vi "Send_picture.vi"() -> ()   [LabVIEW 2018]
uses:
  <vilib>/myRIO/Instrument Drivers/Onboard IO/UART/typedef/VISA Configuration.ctl
  <vilib>/Instr/_visa.llb/VISA Configure Serial Port (Instr).vi
  <vilib>/myRIO/Express VI/Onboard IO/UART/UART Express VI.xnode
  <vilib>/vision/NI_Vision_Development_Module.lvlib
  <vilib>/myRIO/Instrument Drivers/Onboard IO/UART/UART.lvlib
panel:
  out "Picture from local variable":u8[][](graph)
  out "Subarray send.":u8[](array[numeric])
  out "Picture that is send":u8[][](graph)
  out "Length of row":i32
  out "spreadsheet string":string
  out "length of SH string":i32
  in  "File Path":path=path "U:/"
  out "Image Pixels (U8)":u8[][](array[numeric])
  out "Intensity Graph 5":u16[][](graph)
  out "Intensity Graph 3":u8[][](graph)
  out "Original":T1(plugin-control)
  out "Luminance Plane":T1(plugin-control)
  out "Red Plane (as grayscale)":T1(plugin-control)
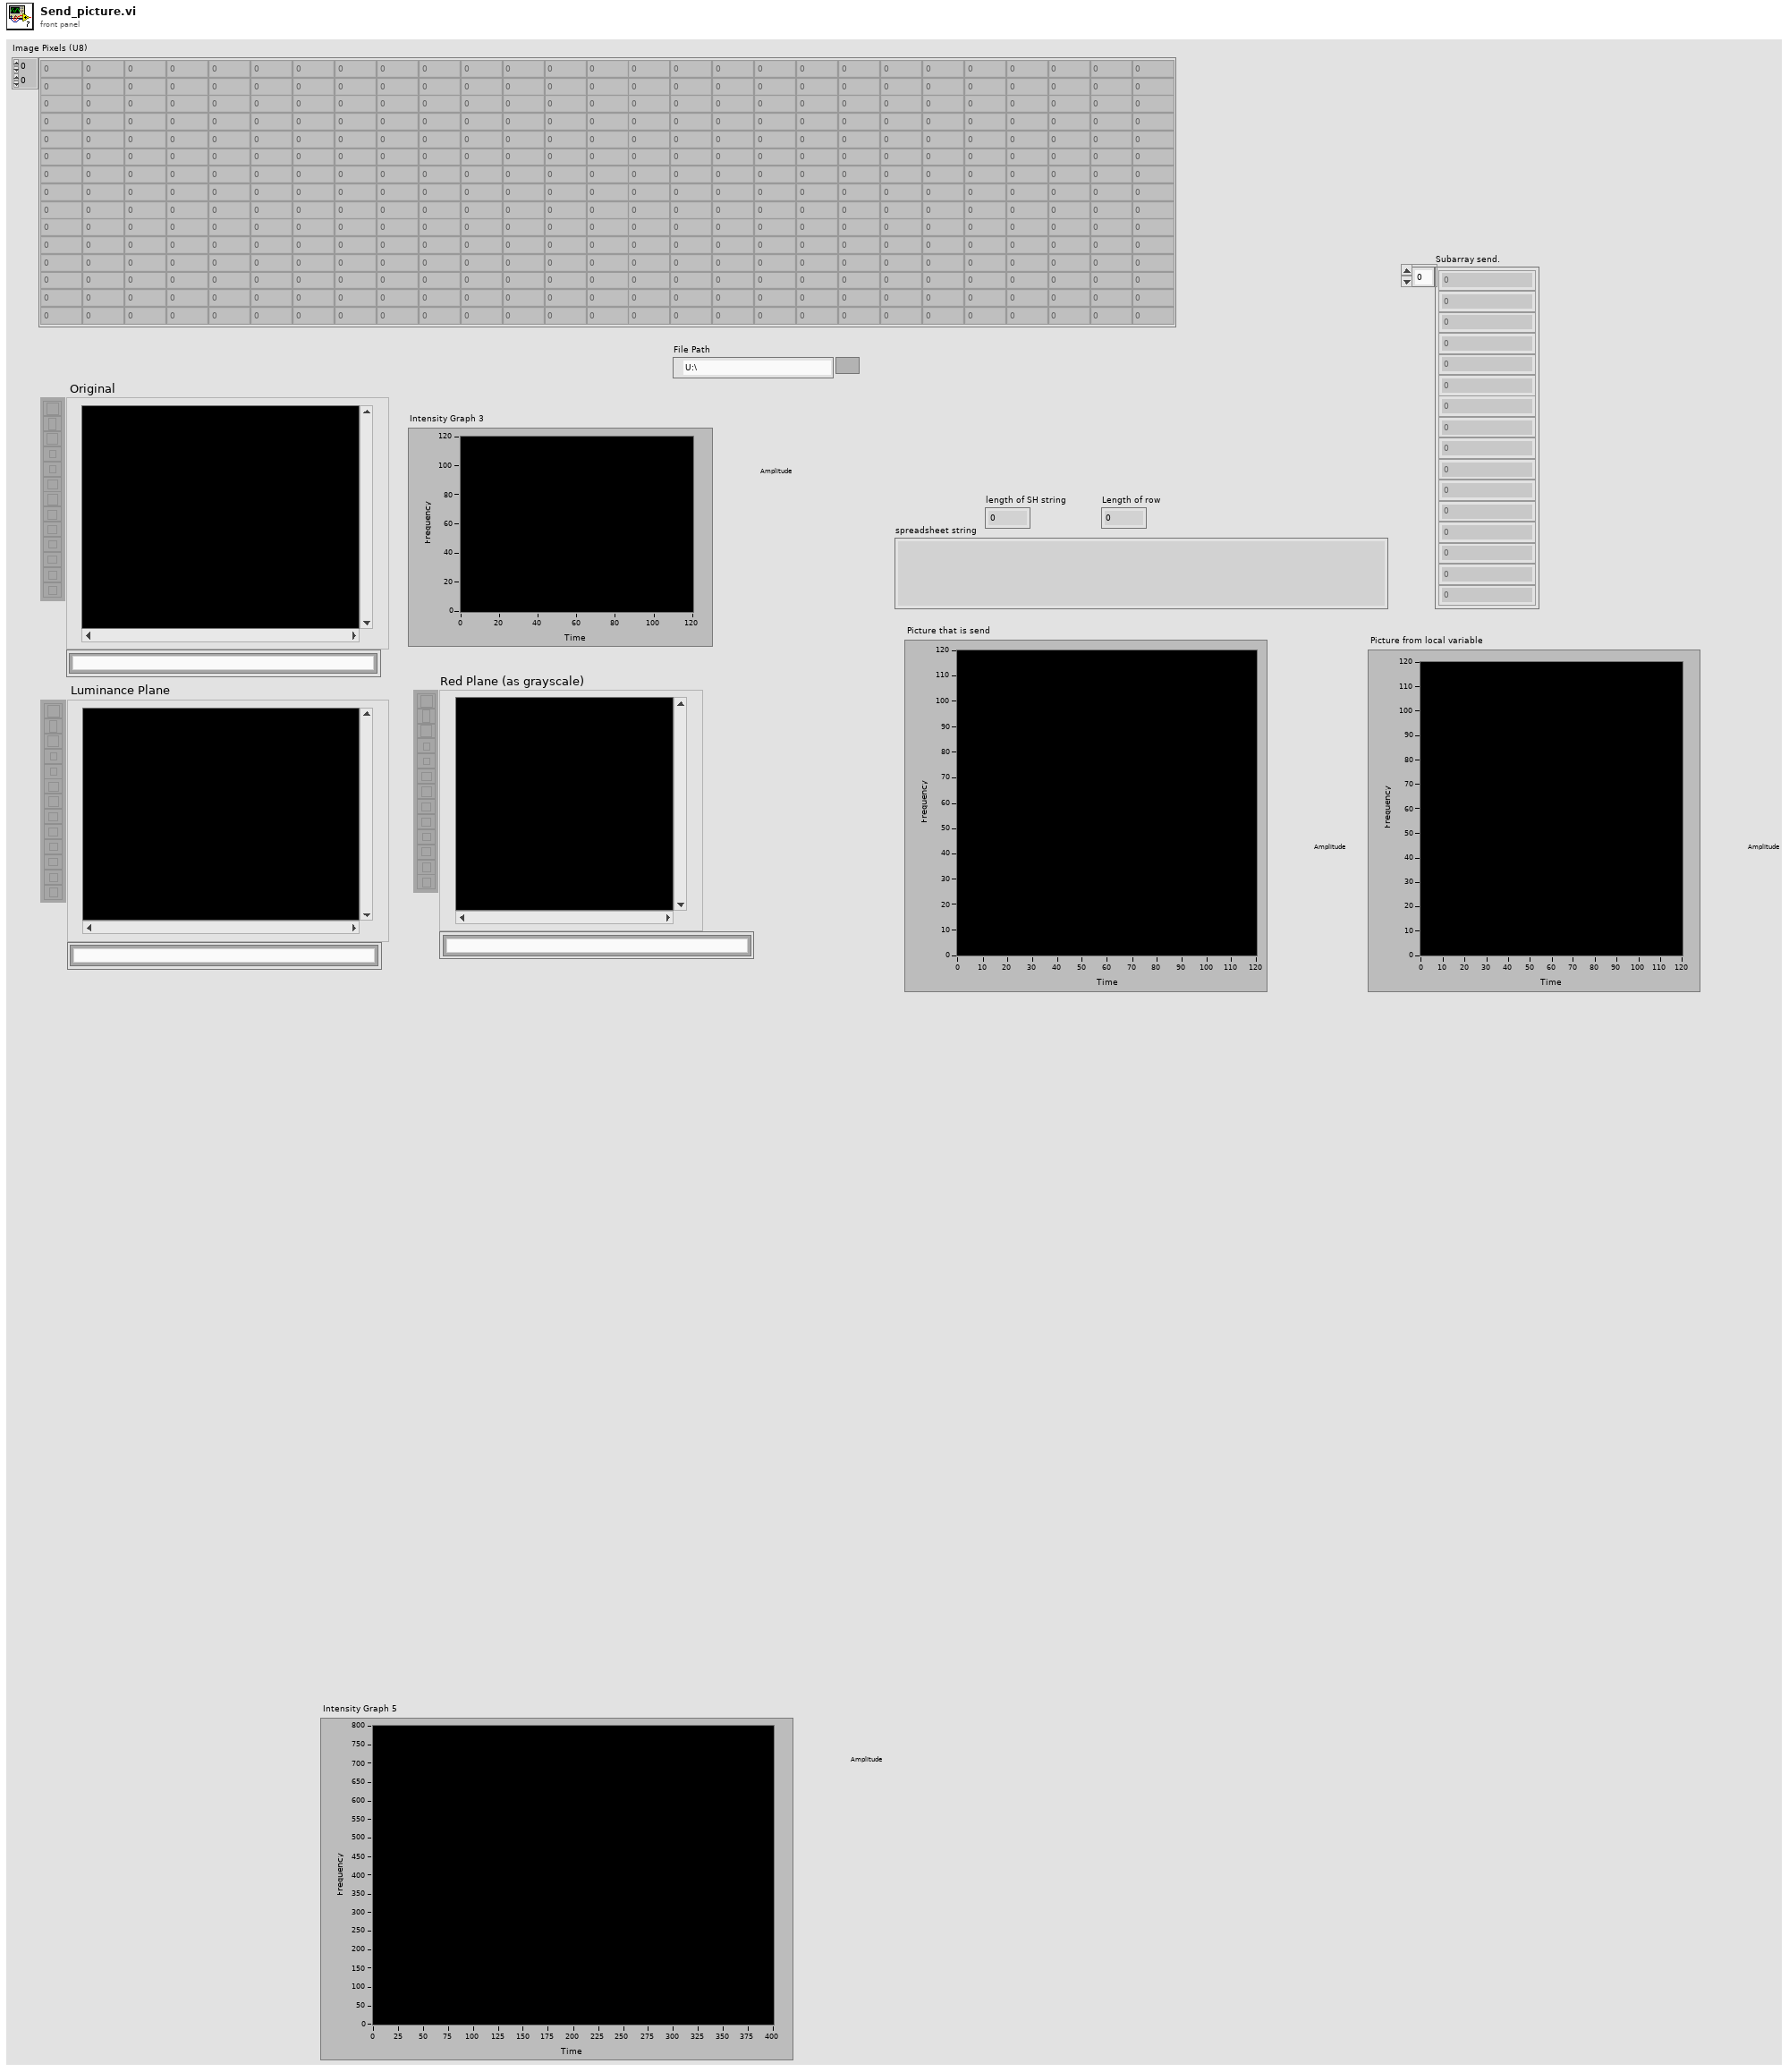
[diagram p1: front panel]
types:
  T1 = typedef "IMAQ Image.ctl" = refnum<image>
  T2 = typedef "Image Type" = u32
  T3 = typedef "UART.lvlib/VISA Configuration.ctl" = cluster{"baud rate (9600)":u32, "data bits (8)":u16, "parity (0:none)":enum16{"None", "Odd", "Even", "Mark", "Space"}, "stop bits (10: 1 bit)":u16, "flow control (0:none)":u16, "termination char\n(0xA = '\\n' = LF) ":u8, "Enable Termination\nChar (T)":bool, "timeout (10sec)":u32}
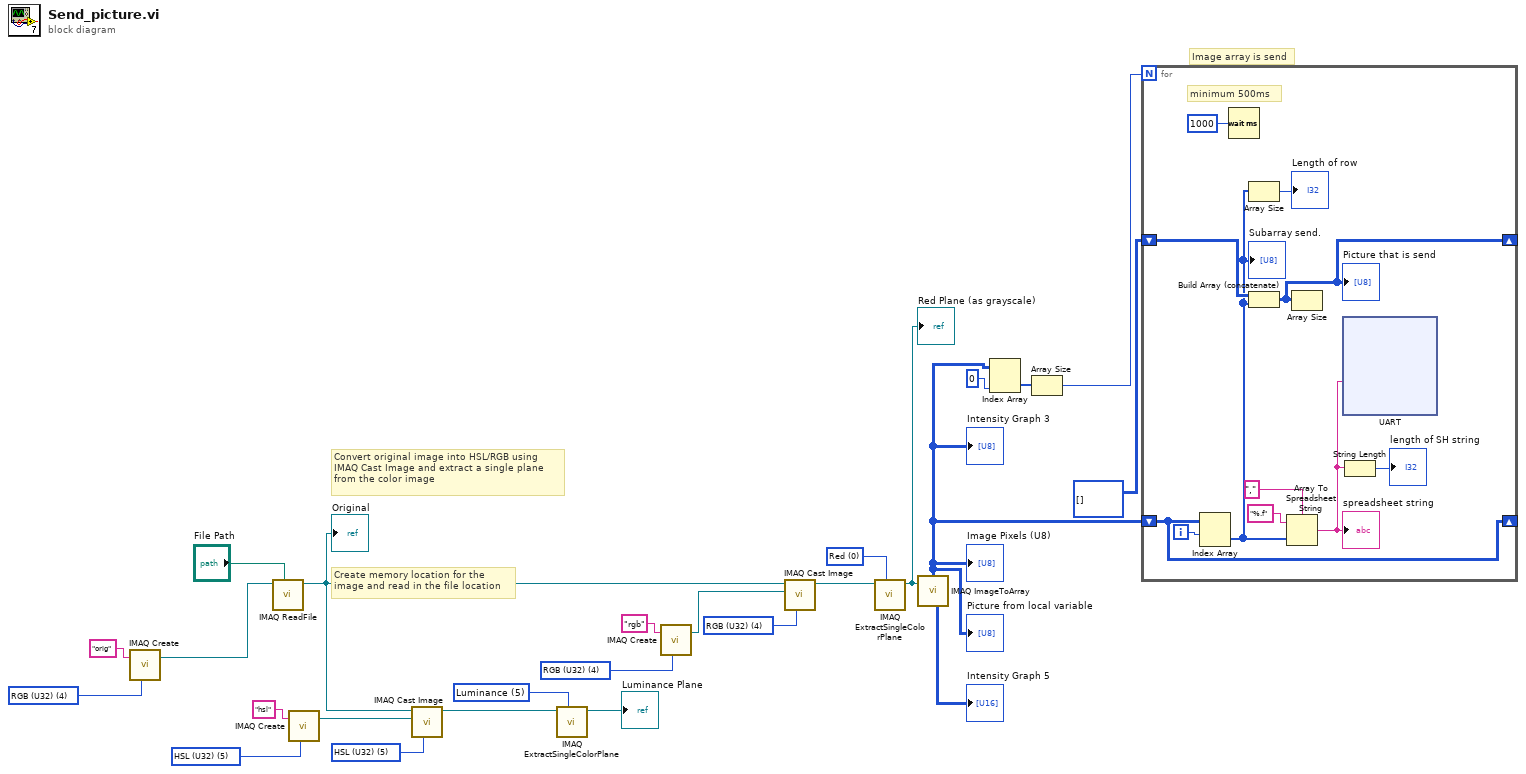
[diagram p0: block diagram]
diagram:
  w22 = T2 4 items=["Grayscale (U8)", "Grayscale (I16)", "Grayscale (SGL)", "Complex (CSG)", "RGB (U32)", "HSL (U32)", "RGB (U64)"] ("Image Type")
  w4 = T2 4 items=["Grayscale (U8)", "Grayscale (I16)", "Grayscale (SGL)", "Complex (CSG)", "RGB (U32)", "HSL (U32)", "RGB (U64)"] ("Image Type")
  w6 = 5 items=["Red", "Green", "Blue", "Hue", "Saturation", "Luminance", "Value", "Intensity"] ("Color Plane")
  w8 = T2 5 items=["Grayscale (U8)", "Grayscale (I16)", "Grayscale (SGL)", "Complex (CSG)", "RGB (U32)", "HSL (U32)", "RGB (U64)"] ("Image Type")
  w9 = T2 5 items=["Grayscale (U8)", "Grayscale (I16)", "Grayscale (SGL)", "Complex (CSG)", "RGB (U32)", "HSL (U32)", "RGB (U64)"] ("Image Type")
  w20 = T2 4 items=["Grayscale (U8)", "Grayscale (I16)", "Grayscale (SGL)", "Complex (CSG)", "RGB (U32)", "HSL (U32)", "RGB (U64)"] ("Image Type")
  w24 = 0 items=["Red", "Green", "Blue", "Hue", "Saturation", "Luminance", "Value", "Intensity"] ("Color Plane")
  # "Convert original image into HSL/RGB using\nIMAQ Cast Image and extract a single plane\nfrom the color image"
  # "Create memory location for the \nimage and read in the file location"
  # "Image array is send"
  n1 = call "IMAQ Create"("Image Name"="orig", "Image Type"=w20) -> ("New Image"=w2:T1)  [unwired: 2 in, 2 out]
  n2 = call "IMAQ ReadFile"("File Path"="File Path", "Image"=w2) -> ("Image Out"=w19:T1)  [unwired: 3 in, 6 out]
  "Original" <- w19
  n3 = call "IMAQ Create"("Image Name"="hsl", "Image Type"=w9) -> ("New Image"=w11:T1)  [unwired: 2 in, 2 out]
  n4 = call "IMAQ Cast Image"("Image Type"=w8, "Image Dst"=w11, "Image Src"=w19) -> ("Image Dst Out"=w7:T1)  [unwired: 3 in, 5 out]
  n5 = call "IMAQ ExtractSingleColorPlane"("Color Plane"=w6, "Image Src"=w7) -> ("Image Dst Out"=→"Luminance Plane":T1)  [unwired: 2 in, 7 out]
  n6 = call "IMAQ Create"("Image Name"="rgb", "Image Type"=w4) -> ("New Image"=w21:T1)  [unwired: 2 in, 2 out]
  n7 = call "IMAQ Cast Image"("Image Type"=w22, "Image Dst"=w21, "Image Src"=w19) -> ("Image Dst Out"=w23:T1)  [unwired: 3 in, 5 out]
  n8 = call "IMAQ ExtractSingleColorPlane"("Color Plane"=w24, "Image Src"=w23) -> ("Image Dst Out"=w18:T1)  [unwired: 2 in, 7 out]
  "Red Plane (as grayscale)" <- w18
  n9 = call "IMAQ ImageToArray"("Image"=w18) -> ("Image Pixels (U16)"=→"Intensity Graph 5":u16[][], "Image Pixels (U8)"=w12:u8[][])  [unwired: 3 in, 3 out]
  "Intensity Graph 3" <- w12
  "Image Pixels (U8)" <- w12
  "Picture from local variable" <- w12
  n10 = Index Array(array=w12, index (col)=0 ("disabled index (col)")) -> (element=w14:u8[])  [unwired: 1 in]
  n11 = Array Size(array=w14) -> (size(s)=w13:i32)
  n12 = for {
    N: w13 -> [_]
    shift-right: [w36] -> _
    shift-left: w12 -> [w36]
    shift-right: [w30] -> _
    shift-left: u8[][] [] -> [w35]
    i -> [w34]
    # "minimum 500ms"
    n13 = Index Array(array=w36, index (row)=w34) -> (element=w28:u8[])  [unwired: 1 in]
    "Subarray send." <- w28
    n14 = Wait (ms)(milliseconds to wait=u32 1000) -> ()  [unwired: 1 out]
    n15 = Array Size(array=w28) -> (size(s)=→"Length of row":i32)
    n16 = Build Array (concatenate)(w35, w28) -> (w30:u8[][])
    "Picture that is send" <- w30
    n17 = Array To Spreadsheet String(delimiter (Tab)=",", array=w28, 3:"%.f" ("format string")) -> (spreadsheet string=w27:string)
    "spreadsheet string" <- w27
    n18 = Array Size(array=w30) -> ()  [unwired: 1 out]
    n19 = xnode "UART"("Characters to Write"=w27) -> ()  [unwired: 1 in, 2 out]
    n20 = String Length(string=w27) -> (length=→"length of SH string":i32)
  }
